vi "Client TCP Core.vi"(8 "error in (no error)":errorcluster, 10 "Command(Params) (\"\")":string, 11 "Client (\"\": localhost)":string) -> (0 "error out":errorcluster, 3 "ACKed Response":string)   [LabVIEW 2011]
uses:
  ITK EXT/http/http0.llb/HTTP LVHTTP Global.vi
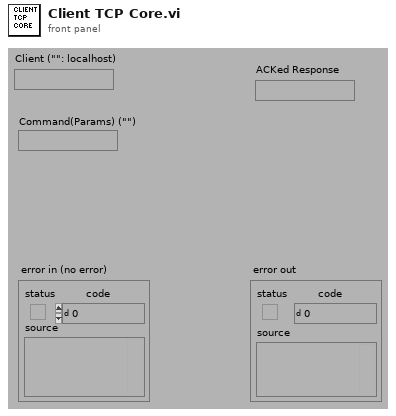
[diagram p1: front panel]
types:
  T1 = enum16{"Standard", "Buffered", "CRLF", "Immediate"}
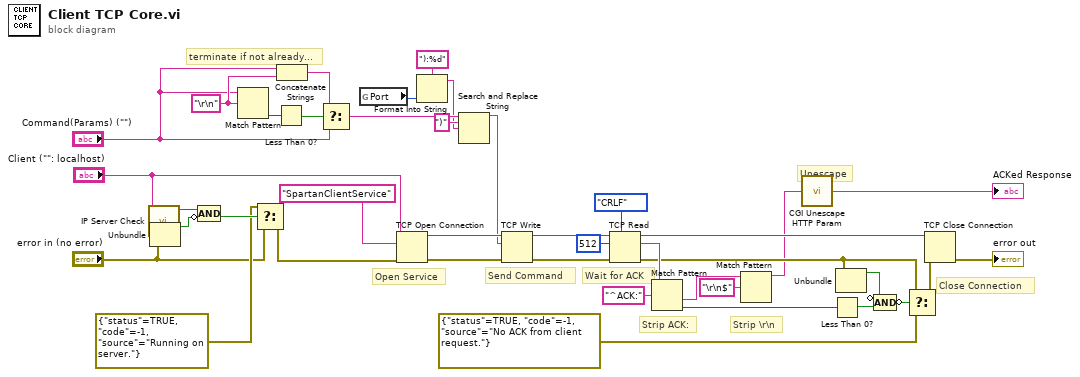
[diagram p0: block diagram]
diagram:
  w13 = "\r\n" ("regular expression")
  # "Unescape"
  # "Strip \\r\\n"
  # "Strip ACK:"
  # "terminate if not already..."
  # "Close Connection"
  # "Wait for ACK"
  # "Send Command"
  # "Open Service"
  n1 = call "IP Server Check.vi"("IP Address"="Client (\"\": localhost)") -> ("IP Same as execution Computer?"=w38:bool)  [unwired: 10 out]
  n2 = Unbundle("error in (no error)") -> ("status"=w37:bool)  [unwired: 2 out]
  n3 = Compound Arithmetic op=AND(w38, invert w37) -> (w36:bool)
  n4 = Match Pattern(string="Command(Params) (\"\")", regular expression=w13) -> (offset past match=w15:i32)  [unwired: 4 out]
  n5 = Select(t=errorcluster {"status"=TRUE, "code"=-1, "source"="Running on server."}, s=w36, f="error in (no error)") -> (s? t:f=w33:errorcluster)
  n6 = Less Than 0?(x=w15) -> (x < 0?=w14:bool)
  n7 = Concatenate Strings("Command(Params) (\"\")", w13) -> (w12:string)
  n8 = Select(t=w12, s=w14, f="Command(Params) (\"\")") -> (s? t:f=w6:string)
  n9 = global read "HTTP LVHTTP Global.vi" "Port"() -> (w3:u16)
  n10 = TCP Open Connection(address="Client (\"\": localhost)", remote port or service name="SpartanClientService", error in (no error)=w33) -> (connection ID=w31:refnum<k5>, error out=w30:errorcluster)  [unwired: 2 out]
  n11 = Format Into String(format string="):%d", w3) -> (resulting string=w2:string)  [unwired: 2 in, 1 out]
  n12 = Search and Replace String(input string=w6, search string=")", replace string=w2) -> (result string=w1:string)  [unwired: 1 in, 7 out]
  n13 = TCP Write(connection ID=w31, data in=w1, error in (no error)=w30) -> (connection ID out=w29:refnum<k5>, error out=w28:errorcluster)  [unwired: 2 out]
  n14 = TCP Read(connection ID=w29, bytes to read=512, error in (no error)=w28, 7:T1."CRLF" ("mode (standard)")) -> (connection ID out=w24:refnum<k5>, data out=w25:string, error out=w18:errorcluster)  [unwired: 1 out]
  n15 = Match Pattern(string=w25, regular expression="^ACK:") -> (after substring=w10:string, offset past match=w22:i32)  [unwired: 3 out]
  n16 = Match Pattern(string=w10, regular expression="\r\n$") -> (before substring=w8:string)  [unwired: 4 out]
  n17 = call "CGI Unescape HTTP Param.vi"("url-encoded string"=w8) -> ("string"=→"ACKed Response":string)
  n18 = Less Than 0?(x=w22) -> (x < 0?=w20:bool)
  n19 = Unbundle(w18) -> ("status"=w19:bool)  [unwired: 2 out]
  n20 = Compound Arithmetic op=AND(invert w19, w20) -> (invert w21:bool)
  n21 = Select(t=w18, s=w21, f=errorcluster {"status"=TRUE, "code"=-1, "source"="No ACK from client request."} ("t")) -> (s? t:f=w17:errorcluster)
  n22 = TCP Close Connection(connection ID=w24, error in (no error)=w17) -> (error out=→"error out":errorcluster)  [unwired: 2 out]
